vi "WS1050 Generate Drives_Command.vi"(8 "error in (no error)":errorcluster, 10 "ALL/UP-DN":bool=TRUE) -> (0 "error out":errorcluster, 2 "Cmd":string[](array[string]), 3 "Driver Name":string[](array[string]))   [LabVIEW 2017]
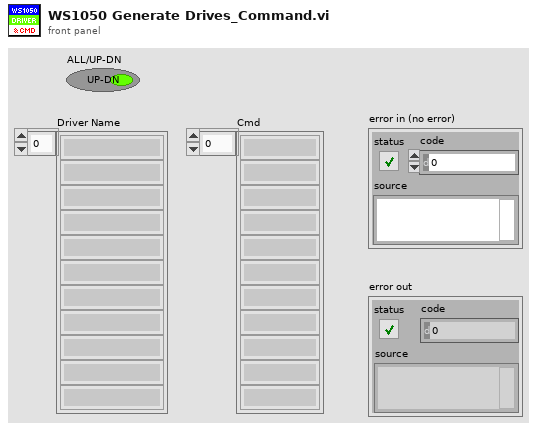
[diagram p1: front panel]
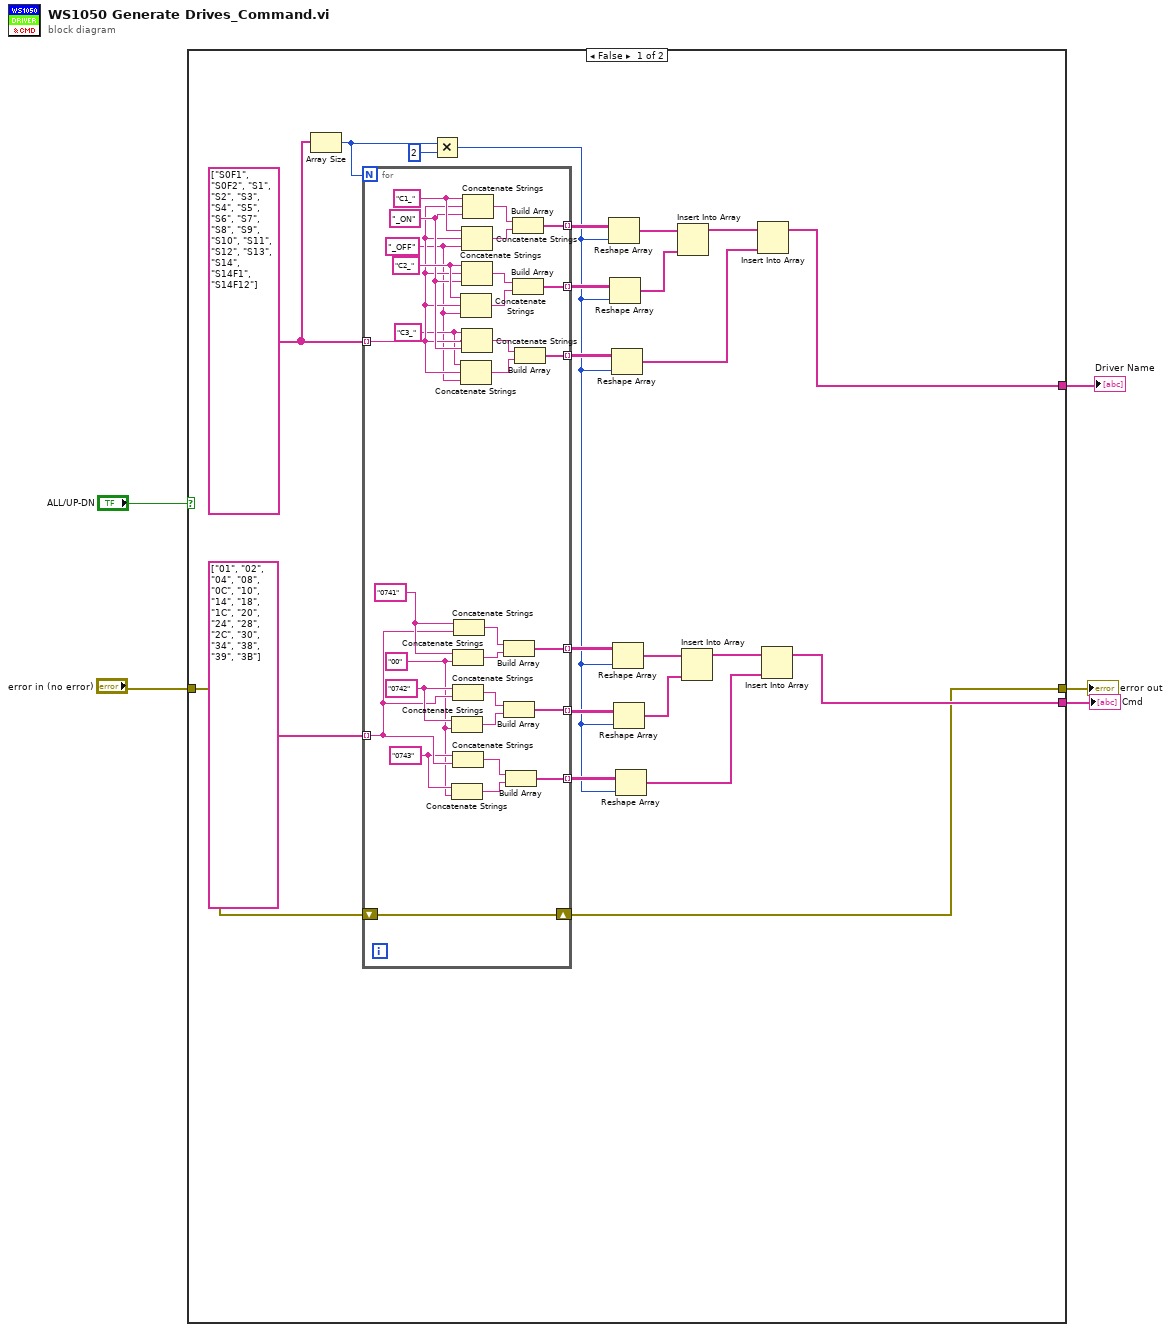
[diagram p0: block diagram]
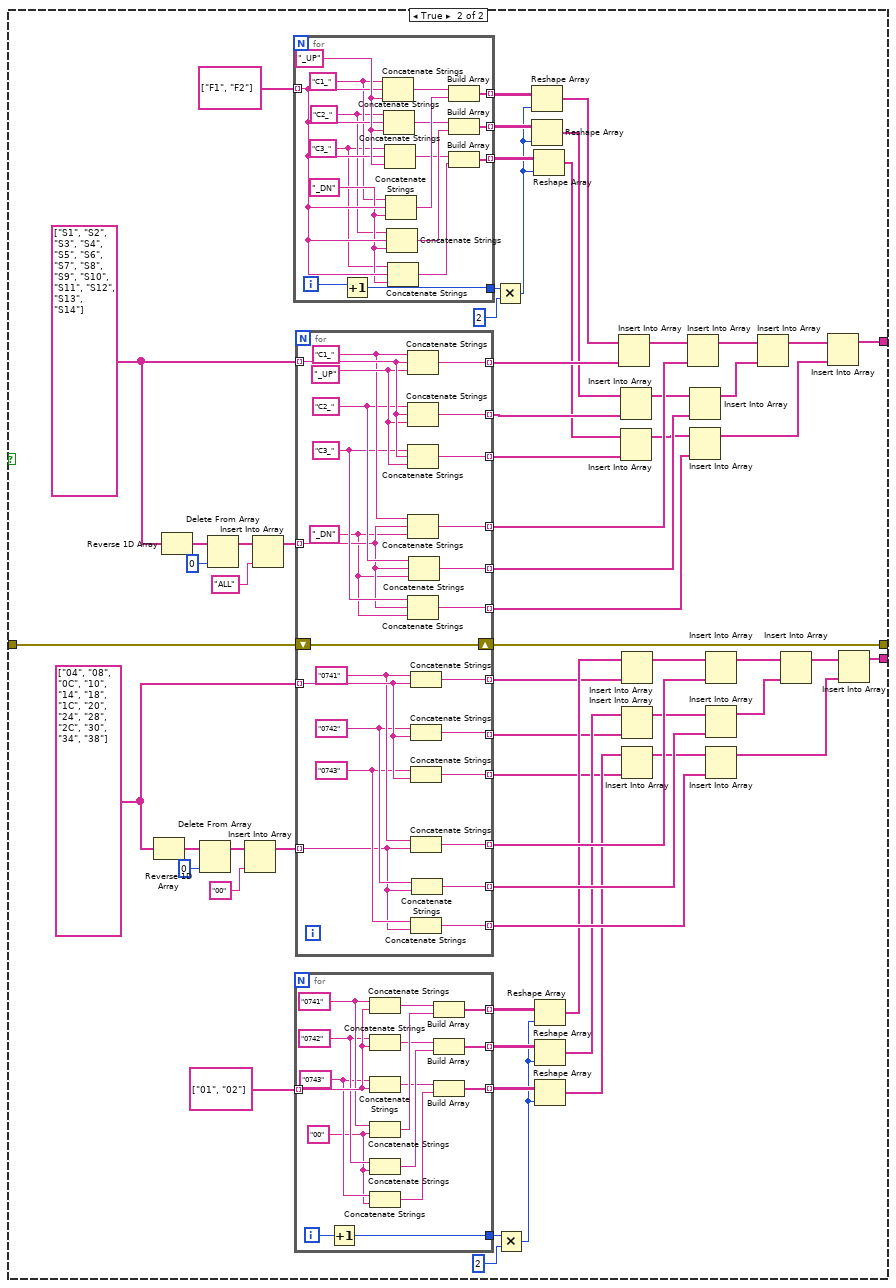
[diagram p2: hidden frame]
diagram:
  n1 = case shown="False" "ALL/UP-DN" {
    tunnel: [w18 w108] -> w5
    tunnel: [w8 w94] -> w4
    tunnel: [w6 w60] -> w2
    tunnel: "error in (no error)" -> [w7 w59]
    frame False {
      w25 = string[] ["S0F1", "S0F2", "S1", "S2", "S3", "S4", "S5", "S6", "S7", "S8", "S9", "S10", "S11", "S12", "S13", "S14", "S14F1", "S14F12"]
      n2 = Array Size(array=w25) -> (size(s)=w24:i32)
      n3 = for {
        N: w24 -> [_]
        tunnel: w25 -> [w53] mode=indexing
        tunnel: [w46] -> w28 mode=indexing
        tunnel: [w45] -> w27 mode=indexing
        tunnel: [w44] -> w26 mode=indexing
        tunnel: string[] ["01", "02", "04", "08", "0C", "10", "14", "18", "1C", "20", "24", "28", "2C", "30", "34", "38", "39", "3B"] -> [w35] mode=indexing
        tunnel: [w32] -> w12 mode=indexing
        tunnel: [w31] -> w11 mode=indexing
        tunnel: [w30] -> w10 mode=indexing
        shift-right: [w29] -> w6
        shift-left: w7 -> [w29]
        w34 = "0743" ("string")
        w36 = "0742" ("string")
        w33 = "00" ("string")
        w37 = "0741" ("string")
        w52 = "C3_" ("string")
        w55 = "C2_" ("string")
        w51 = "_OFF" ("string")
        w54 = "_ON" ("string")
        w58 = "C1_" ("string")
        n4 = Concatenate Strings(w36, w33) -> (w43:string)
        n5 = Concatenate Strings(w34, w33) -> (w41:string)
        n6 = Concatenate Strings(w37, w33) -> (w39:string)
        n7 = Concatenate Strings(w36, w35) -> (w42:string)
        n8 = Concatenate Strings(w34, w35) -> (w40:string)
        n9 = Concatenate Strings(w37, w35) -> (w38:string)
        n10 = Concatenate Strings(w55, w53, w51) -> (w47:string)
        n11 = Concatenate Strings(w52, w53, w51) -> (w49:string)
        n12 = Concatenate Strings(w58, w53, w51) -> (w56:string)
        n13 = Concatenate Strings(w55, w53, w54) -> (w48:string)
        n14 = Concatenate Strings(w52, w53, w54) -> (w50:string)
        n15 = Concatenate Strings(w58, w53, w54) -> (w57:string)
        n16 = Build Array(w38, w39) -> (w32:string[])
        n17 = Build Array(w42, w43) -> (w31:string[])
        n18 = Build Array(w40, w41) -> (w30:string[])
        n19 = Build Array(w57, w56) -> (w46:string[])
        n20 = Build Array(w48, w47) -> (w45:string[])
        n21 = Build Array(w50, w49) -> (w44:string[])
      }
      n22 = Multiply(x=w24, y=2) -> (x*y=w9:i32)
      n23 = Reshape Array(w28, w9) -> (w22:string[])
      n24 = Reshape Array(w27, w9) -> (w21:string[])
      n25 = Reshape Array(w26, w9) -> (w20:string[])
      n26 = Reshape Array(w12, w9) -> (w13:string[])
      n27 = Reshape Array(w11, w9) -> (w14:string[])
      n28 = Reshape Array(w10, w9) -> (w15:string[])
      n29 = Insert Into Array(array=w22, new element=w21) -> (w19:string[])  [unwired: 1 in]
      n30 = Insert Into Array(array=w13, new element=w14) -> (w16:string[])  [unwired: 1 in]
      n31 = Insert Into Array(array=w19, new element=w20) -> (w18:string[])  [unwired: 1 in]
      n32 = Insert Into Array(array=w16, new element=w15) -> (w8:string[])  [unwired: 1 in]
    }
    frame True {
      w105 = string[] ["04", "08", "0C", "10", "14", "18", "1C", "20", "24", "28", "2C", "30", "34", "38"]
      w93 = string[] ["S1", "S2", "S3", "S4", "S5", "S6", "S7", "S8", "S9", "S10", "S11", "S12", "S13", "S14"]
      n33 = Reverse 1D Array(array=w105) -> (reversed array=w104:string[])
      n34 = Reverse 1D Array(array=w93) -> (reversed array=w120:string[])
      n35 = Delete From Array(array=w104, index=0) -> (array with subset deleted=w103:string[])  [unwired: 1 in, 1 out]
      n36 = Delete From Array(array=w120, index=0) -> (array with subset deleted=w118:string[])  [unwired: 1 in, 1 out]
      n37 = Insert Into Array(array=w103, new element="00" ("new element/subarray")) -> (w102:string[])  [unwired: 1 in]
      n38 = Insert Into Array(array=w118, new element="ALL" ("new element/subarray")) -> (w116:string[])  [unwired: 1 in]
      n39 = for {
        tunnel: string[] ["F1", "F2"] -> [w152] mode=indexing
        tunnel: [w143] -> w91 mode=indexing
        tunnel: [w146] -> w79
        tunnel: [w140] -> w87 mode=indexing
        tunnel: [w137] -> w83 mode=indexing
        i -> [w147]
        w151 = "_DN" ("string")
        w148 = "C3_" ("string")
        w149 = "C2_" ("string")
        w153 = "_UP" ("string")
        w150 = "C1_" ("string")
        n40 = Increment(x=w147) -> (x+1=w146:i32)
        n41 = Concatenate Strings(w150, w152, w153) -> (w144:string)
        n42 = Concatenate Strings(w149, w152, w153) -> (w142:string)
        n43 = Concatenate Strings(w148, w152, w153) -> (w139:string)
        n44 = Concatenate Strings(w150, w152, w151) -> (w145:string)
        n45 = Concatenate Strings(w149, w152, w151) -> (w141:string)
        n46 = Concatenate Strings(w148, w152, w151) -> (w138:string)
        n47 = Build Array(w144, w145) -> (w143:string[])
        n48 = Build Array(w142, w141) -> (w140:string[])
        n49 = Build Array(w139, w138) -> (w137:string[])
      }
      n50 = for {
        tunnel: string[] ["01", "02"] -> [w136] mode=indexing
        tunnel: [w125] -> w73 mode=indexing
        tunnel: [w124] -> w72 mode=indexing
        tunnel: [w123] -> w71 mode=indexing
        tunnel: [w121] -> w75
        i -> [w122]
        w132 = "00" ("string")
        w133 = "0743" ("string")
        w134 = "0742" ("string")
        w135 = "0741" ("string")
        n51 = Increment(x=w122) -> (x+1=w121:i32)
        n52 = Concatenate Strings(w135, w136) -> (w131:string)
        n53 = Concatenate Strings(w134, w136) -> (w129:string)
        n54 = Concatenate Strings(w133, w136) -> (w127:string)
        n55 = Concatenate Strings(w135, w132) -> (w130:string)
        n56 = Concatenate Strings(w134, w132) -> (w128:string)
        n57 = Concatenate Strings(w133, w132) -> (w126:string)
        n58 = Build Array(w131, w130) -> (w125:string[])
        n59 = Build Array(w129, w128) -> (w124:string[])
        n60 = Build Array(w127, w126) -> (w123:string[])
      }
      n61 = for {
        tunnel: w93 -> [w178] mode=indexing
        tunnel: w116 -> [w173] mode=indexing
        tunnel: [w171] -> w90 mode=indexing
        tunnel: [w170] -> w115 mode=indexing
        tunnel: [w169] -> w85 mode=indexing
        tunnel: [w168] -> w114 mode=indexing
        tunnel: [w167] -> w82 mode=indexing
        tunnel: [w166] -> w113 mode=indexing
        tunnel: w105 -> [w165] mode=indexing
        tunnel: w102 -> [w161] mode=indexing
        tunnel: [w160] -> w68 mode=indexing
        tunnel: [w159] -> w66 mode=indexing
        tunnel: [w158] -> w63 mode=indexing
        tunnel: [w157] -> w97 mode=indexing
        tunnel: [w156] -> w96 mode=indexing
        tunnel: [w155] -> w95 mode=indexing
        shift-right: [w154] -> w60
        shift-left: w59 -> [w154]
        w162 = "0743" ("string")
        w163 = "0742" ("string")
        w164 = "0741" ("string")
        w172 = "_DN" ("string")
        w174 = "C3_" ("string")
        w175 = "C2_" ("string")
        w177 = "_UP" ("string")
        w176 = "C1_" ("string")
        n62 = Concatenate Strings(w176, w178, w177) -> (w171:string)
        n63 = Concatenate Strings(w175, w178, w177) -> (w169:string)
        n64 = Concatenate Strings(w174, w178, w177) -> (w167:string)
        n65 = Concatenate Strings(w176, w173, w172) -> (w170:string)
        n66 = Concatenate Strings(w174, w173, w172) -> (w166:string)
        n67 = Concatenate Strings(w175, w173, w172) -> (w168:string)
        n68 = Concatenate Strings(w164, w165) -> (w160:string)
        n69 = Concatenate Strings(w163, w165) -> (w159:string)
        n70 = Concatenate Strings(w162, w165) -> (w158:string)
        n71 = Concatenate Strings(w164, w161) -> (w157:string)
        n72 = Concatenate Strings(w162, w161) -> (w155:string)
        n73 = Concatenate Strings(w163, w161) -> (w156:string)
      }
      n74 = Multiply(x=w79, y=2) -> (x*y=w78:i32)
      n75 = Multiply(x=w75, y=2) -> (x*y=w61:i32)
      n76 = Reshape Array(w91, w78) -> (w88:string[])
      n77 = Reshape Array(w87, w78) -> (w84:string[])
      n78 = Reshape Array(w83, w78) -> (w81:string[])
      n79 = Reshape Array(w73, w61) -> (w69:string[])
      n80 = Reshape Array(w72, w61) -> (w67:string[])
      n81 = Reshape Array(w71, w61) -> (w64:string[])
      n82 = Insert Into Array(array=w88, new element=w90) -> (w89:string[])  [unwired: 1 in]
      n83 = Insert Into Array(array=w84, new element=w85) -> (w86:string[])  [unwired: 1 in]
      n84 = Insert Into Array(array=w81, new element=w82) -> (w80:string[])  [unwired: 1 in]
      n85 = Insert Into Array(array=w69, new element=w68) -> (w70:string[])  [unwired: 1 in]
      n86 = Insert Into Array(array=w67, new element=w66) -> (w65:string[])  [unwired: 1 in]
      n87 = Insert Into Array(array=w64, new element=w63) -> (w62:string[])  [unwired: 1 in]
      n88 = Insert Into Array(array=w89, new element=w115) -> (w112:string[])  [unwired: 1 in]
      n89 = Insert Into Array(array=w86, new element=w114) -> (w111:string[])  [unwired: 1 in]
      n90 = Insert Into Array(array=w80, new element=w113) -> (w109:string[])  [unwired: 1 in]
      n91 = Insert Into Array(array=w70, new element=w97) -> (w98:string[])  [unwired: 1 in]
      n92 = Insert Into Array(array=w65, new element=w96) -> (w99:string[])  [unwired: 1 in]
      n93 = Insert Into Array(array=w62, new element=w95) -> (w101:string[])  [unwired: 1 in]
      n94 = Insert Into Array(array=w112, new element=w111) -> (w110:string[])  [unwired: 1 in]
      n95 = Insert Into Array(array=w98, new element=w99) -> (w100:string[])  [unwired: 1 in]
      n96 = Insert Into Array(array=w110, new element=w109) -> (w108:string[])  [unwired: 1 in]
      n97 = Insert Into Array(array=w100, new element=w101) -> (w94:string[])  [unwired: 1 in]
    }
  }
  "Driver Name" <- w5
  "Cmd" <- w4
  "error out" <- w2
